vi "Initialize or Close Instrument Sessions.vi"(0 "TSM Context":T1, 5 "Operation":enum16{"Initialize", "Close"}(ring), 11 "error in":errorcluster) -> (15 "error out":errorcluster)   [LabVIEW 2023]
uses:
  <vilib>/NI_TestStand_SemiconductorModule/NI_TestStand_Semiconductor_Module.lvlibp/PinMap/General/SemiconductorModuleContext.ctl
  <vilib>/NI_TestStand_SemiconductorModule/NI_TestStand_Semiconductor_Module.lvlibp
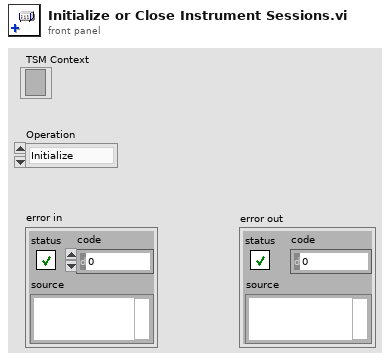
[diagram p1: front panel]
types:
  T1 = typedef "NI_TestStand_Semiconductor_Module.lvlibp/SemiconductorModuleContext.ctl" = refnum<k7>
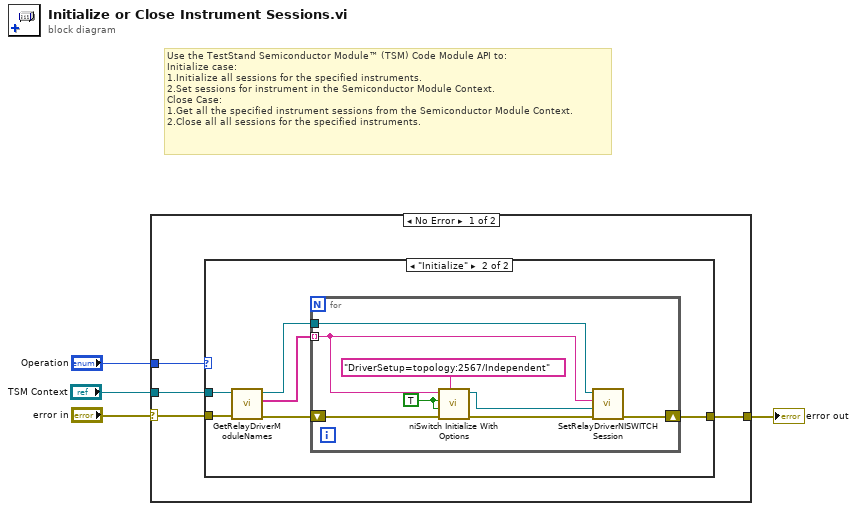
[diagram p0: block diagram]
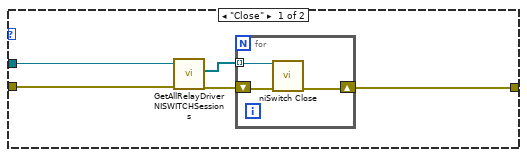
[diagram p2: hidden frame]
diagram:
  # "Use the TestStand Semiconductor Module™ (TSM) Code Module API to:\nInitialize case:\n1.Initialize all sessions for the specified instruments.\n2.Set sessions for instrument in the Semiconductor Module Context.\nClose Case:\n1.Get all the specified instrument sessions from the Semiconductor Module Context.\n2.Close all all sessions for the specified instruments."
  n1 = case shown="No Error" "error in" {
    selector: "error in" -> [w8 w31]
    tunnel: "TSM Context" -> [w7 _]
    tunnel: "Operation" -> [w6 _]
    tunnel: [w5 w31] -> w1
    frame No Error {
      n2 = case shown="\"Initialize\"" w6 {
        tunnel: w8 -> [w11 w22]
        tunnel: w7 -> [w9 w21]
        tunnel: [w10 w17] -> w5
        frame "Close" {
          n3 = call <vilib>:"GetAllRelayDriverNISWITCHSessions.vi"("error in (no error)"=w11, "Semiconductor Module Context"=w9) -> ("error out"=w12:errorcluster, "NI-SWITCH Sessions"=w13:refnum<k15>[])  [unwired: 7 in, 1 out]
          n4 = for {
            tunnel: w13 -> [w14] mode=indexing
            shift-right: [w16] -> w10
            shift-left: w12 -> [w15]
            n5 = call <instrlib>:"niSwitch Close.vi"("error in (no error)"=w15, "instrument handle"=w14) -> ("error out"=w16:errorcluster)  [unwired: 9 in]
          }
        }
        frame "Initialize" {
          n6 = call <vilib>:"GetRelayDriverModuleNames.vi"("error in (no error)"=w22, "Semiconductor Module Context"=w21) -> ("error out"=w20:errorcluster, "Module Names"=w19:string[], "Semiconductor Module Context Out"=w18:T1)  [unwired: 7 in]
          n7 = for {
            shift-right: [w30] -> w17
            shift-left: w20 -> [w28]
            tunnel: w19 -> [w23] mode=indexing
            tunnel: w18 -> [w24]
            w27 = TRUE ("id query (boolean value)")
            n8 = call <instrlib>:"niSwitch Initialize With Options.vi"("option string (Simulate=0,RangeCheck=1,DriverSetup=topology:1127/2-Wire 32x1 Mux)"="DriverSetup=topology:2567/Independent" ("option string (Simulate=0,RangeCheck=1,DriverSetup=topology:1127/2-Wire 32x1 Mux)"), "error in (no error)"=w28, "reset device (boolean value)"=w27, "id query (boolean value)"=w27, "resource name"=w23) -> ("error out"=w29:errorcluster, "instrument handle out"=w25:refnum<k15>)  [unwired: 5 in]
            n9 = call <vilib>:"SetRelayDriverNISWITCHSession.vi"("error in (no error)"=w29, "NI-SWITCH Session"=w25, "Relay Driver Module Name"=w23, "Semiconductor Module Context"=w24) -> ("error out"=w30:errorcluster)  [unwired: 6 in, 1 out]
          }
        }
      }
    }
    frame Error {
    }
  }
  "error out" <- w1
